vi "PCA9525 - GMON.vi"(8 "error in (no error)":errorcluster, 10 "buffer":u8[](array[numeric])=[2, 255, 255], 11 "handle":u64 format="%x") -> (0 "error out":errorcluster, 1 "p/f4":bool, 3 "handle out":u64)   [LabVIEW 2024]
doc: "Control on eSTOP on RIB Tickler\nAll relay are set to an output then a buffer can be edited to control which relays are high and low."
panel:
  out "sizeTransferred 2":u32
  out "sizeTransferred (Output) 2":u32
  out "sizeTransferred (Output)":u32
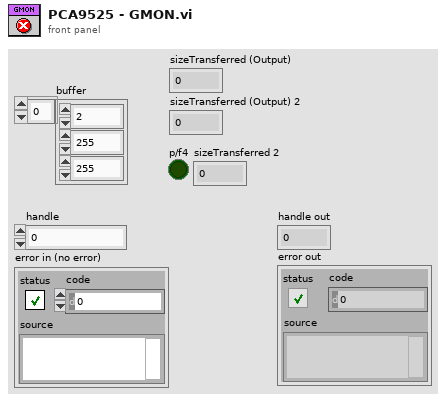
[diagram p1: front panel]
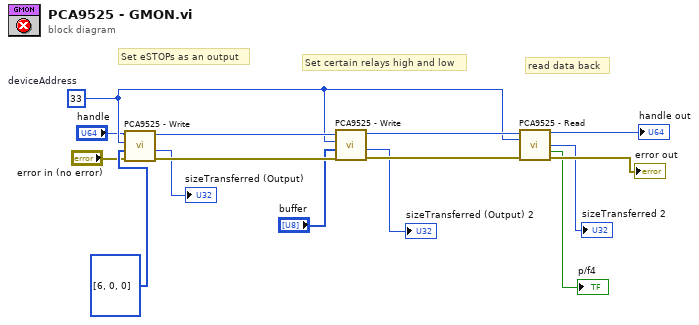
[diagram p0: block diagram]
diagram:
  w9 = u8 33  # deviceAddress
  # "read data back"
  # "Set certain relays high and low"
  # "Set eSTOPs as an output"
  n1 = call "PCA9525 - Write.vi"("error in (no error)"="error in (no error)", "buffer"=u8[] [6, 0, 0], "deviceAddress"=w9, "handle"="handle") -> ("error out"=w14:errorcluster, "sizeTransferred (Output)"=→"sizeTransferred (Output)":u32, "handle 2"=w15:u64)  [unwired: 4 in, 1 out]
  n2 = call "PCA9525 - Write.vi"("error in (no error)"=w14, "buffer"="buffer", "deviceAddress"=w9, "handle"=w15) -> ("error out"=w11:errorcluster, "sizeTransferred (Output)"=→"sizeTransferred (Output) 2":u32, "handle 2"=w13:u64)  [unwired: 4 in, 1 out]
  n3 = call "PCA9525 - Read.vi"("Handle In"=w13, "deviceAddress"=w9, "error in (no error)"=w11) -> ("handle"=→"handle out":u64, "sizeTransferred"=→"sizeTransferred 2":u32, "pass?"=→"p/f4":bool, "error out"=→"error out":errorcluster)  [unwired: 8 in, 1 out]
